vi "NI6602.ProcPeriodic.vi"(0 "i ref in":refnum<vi>, 3 "ms timeout (10000)":i32=10000, 5 "error in (no error)":errorcluster) -> (14 "i ref out":refnum<vi>, 17 "timed out":bool, 19 "error out":errorcluster)   [LabVIEW 2014, in "NI6602.lvlib"]
doc: "This method serves to periodically do things like reading values from the HW. Methods that should be executed periodically should be called from THIS methode. Add code here."
uses:
  NI6602.lvlib
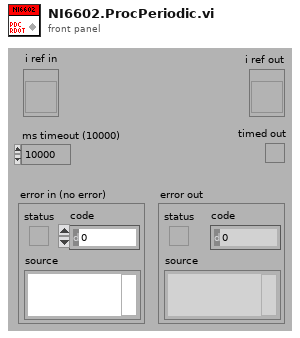
[diagram p1: front panel]
types:
  T1 = typedef "NI6602.lvlib/NI6602.i attribute.ctl" = cluster{"CounterDAQ Channels":cluster{"task":refnum<k21>, "Channel Name":string}[], "RateServiceIDs":i32[], "Running?":bool, "IntegralServiceIDs":i32[], "ThresholdID":i32, "Threshold":dbl, "IntegralValues":dbl[], "Stopped?":bool}
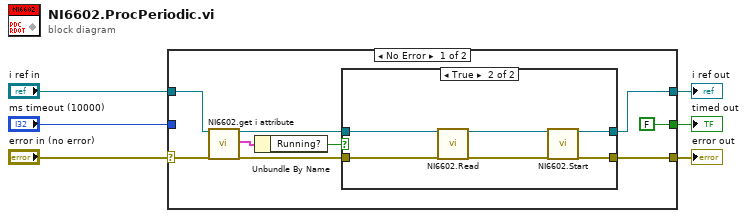
[diagram p0: block diagram]
diagram:
  n1 = case shown="No Error" "error in (no error)" {
    selector: "error in (no error)" -> [w14 w24]
    tunnel: [w8 w24] -> w5
    tunnel: "i ref in" -> [w13 w25]
    tunnel: [w7 w25] -> w3
    tunnel: [FALSE _] -> w2
    tunnel: "ms timeout (10000)" -> [_ _]
    frame No Error {
      n2 = call "NI6602.get i attribute.vi"("i ref in"=w13, "error in (no error)"=w14) -> ("i ref out"=w9:refnum<vi>, "i attribute"=w12:T1, "error out"=w10:errorcluster)  [unwired: 15 in]
      n3 = Unbundle By Name(w12) -> ("Running?"=w11:bool)
      n4 = case shown="True" w11 {
        tunnel: w10 -> [w16 w22]
        tunnel: w9 -> [w17 w23]
        tunnel: [w16 w19] -> w8
        tunnel: [w17 w18] -> w7
        frame False {
        }
        frame True {
          n5 = call "NI6602.Read.vi"("i ref in"=w23, "error in (no error)"=w22) -> ("i ref out"=w21:refnum<vi>, "error out"=w20:errorcluster)  [unwired: 16 in]
          n6 = call "NI6602.Start.vi"("i ref in"=w21, "error in (no error)"=w20) -> ("i ref out"=w18:refnum<vi>, "error out"=w19:errorcluster)  [unwired: 16 in]
        }
      }
    }
    frame Error {
    }
  }
  "error out" <- w5
  "i ref out" <- w3
  "timed out" <- w2
